vi "Comms Main.vi"(8 "error in (no error)":errorcluster, 11 "UDP Ref":refnum<k16>) -> (0 "error out":errorcluster, 3 "UDP Ref Out":refnum<k16>)   [LabVIEW 2019]
uses:
  Application Support/Stop Button/SubVI/Get Stop Button Status.vi
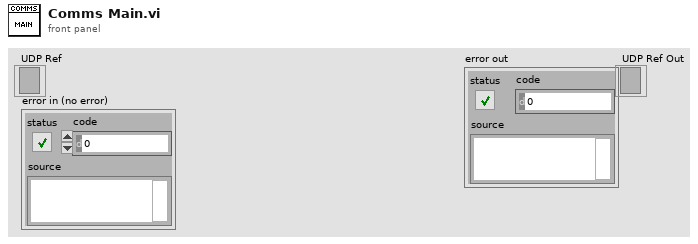
[diagram p1: front panel]
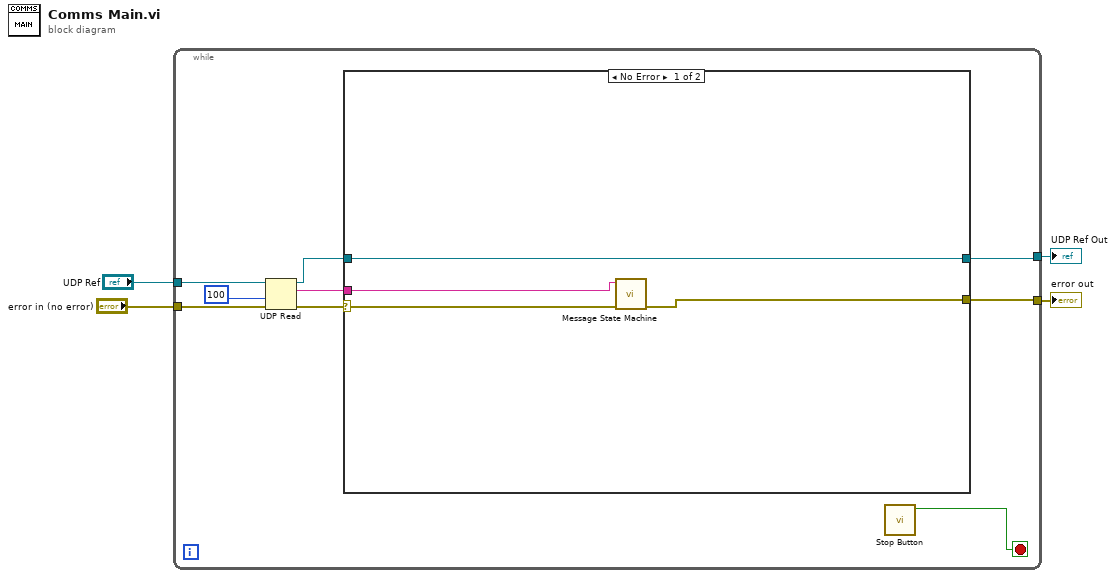
[diagram p0: block diagram]
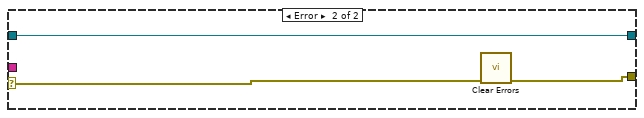
[diagram p2: hidden frame]
diagram:
  n1 = while {
    tunnel: "UDP Ref" -> [w12]
    tunnel: "error in (no error)" -> [w11]
    tunnel: [w7] -> w2
    tunnel: [w6] -> w1
    stop <- w10 stop-if-true
    n2 = UDP Read(connection ID=w12, timeout ms (25000)=100, 8:w11) -> (data out=w8:string, error out=w9:errorcluster, 3:w5:refnum<k16>)  [unwired: 3 out]
    n3 = case shown="No Error" w9 {
      selector: w9 -> [w17 w19]
      tunnel: w8 -> [w16 _]
      tunnel: [w15 w20] -> w7
      tunnel: [w14 w18] -> w6
      tunnel: w5 -> [w14 w18]
      frame No Error {
        n4 = call "Message State Machine.vi"("error in (no error)"=w17, "Message"=w16) -> ("error out"=w15:errorcluster)  [unwired: 9 in]
      }
      frame Error {
        n5 = call <vilib>:"Clear Errors.vi"("error in (no error)"=w19) -> ("error out"=w20:errorcluster)  [unwired: 5 in, 1 out]
      }
    }
    n6 = call-poly "Stop Button.vi"() -> ("Stop ButtonOut"=w10:bool)  [unwired: 10 in, 1 out]
  }
  "error out" <- w2
  "UDP Ref Out" <- w1
